vi "testbeep.vi"   [LabVIEW 2015]
uses:
  G_ALL.vi
types:
  T1 = cluster{"beep":bool, "duration (msec)":u32, "frequency (Hz)":u32}
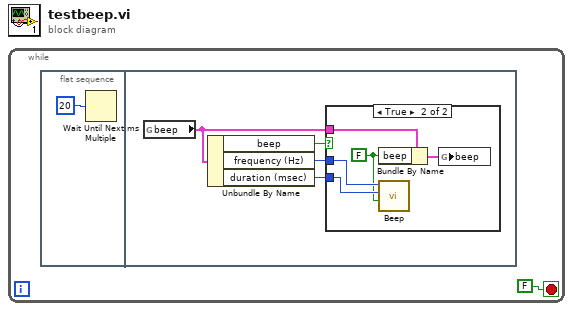
[diagram p0: block diagram]
diagram:
  n1 = while {
    stop <- FALSE stop-if-true
    n2 = flat-sequence {
      frame #0 {
        n3 = Wait Until Next ms Multiple(millisecond multiple=u32 20 ("millisecond timer value")) -> ()  [unwired: 1 out]
      }
      frame #1 {
        n4 = global read "G_ALL.vi" "beep"() -> (w3:T1)
        n5 = Unbundle By Name(w3) -> ("beep"=w6:bool, "frequency (Hz)"=w5:u32, "duration (msec)"=w4:u32)
        n6 = case shown="True" w6 {
          tunnel: w5 -> [_ w11]
          tunnel: w4 -> [_ w10]
          tunnel: w3 -> [_ w7]
          frame False {
          }
          frame True {
            w9 = FALSE ("use system alert? (T)")
            n7 = Bundle By Name(cluster=w7, "beep"=w9) -> (w8:T1)
            n8 = call <vilib>:"Beep.vi"("use system alert? (T)"=w9, "duration (msec)"=w10, "frequency (Hz)"=w11) -> ()  [unwired: 9 in]
            n9 = global write "G_ALL.vi" "beep"(w8) -> ()
          }
        }
      }
    }
  }
